vi "Untitled 9 (SubVI).vi"(0 "background \n coincidence counts":dbl, 1 "sigma (mrad) in":dbl, 2 "collimator afstand\n       (mm)":dbl, 3 "alignment correction":dbl, 4 "spleetbreedte\n      (mm)":dbl, 5 "1d - Acar":bool, 6 "all rows":ext[][](array[numeric]), 8 "22Na source radius (mm)":dbl, 9 "stop in":bool, 10 "core width\n   (mrad)":dbl, 11 "stop 4":bool, 12 "fraction core\nannihilations":dbl, 14 "Fermi angle\n   (mrad)":dbl) -> (13 "2d - Acar 4":bool, 15 "2d - Acar 2":bool, 16 "free gas model":cluster{"Y":dbl[], "Y":dbl[]}[](graph), 17 "ZICHT  functie":cluster{"Y":dbl[], "Y":dbl[]}[](graph), 18 "core electrons":cluster{"Y":dbl[], "Y":dbl[]}[](graph), 19 "2d - Acar 3":bool, 20 "output cluster 2":cluster{ext[], ext[]}, 21 "Sum of squared residuals":dbl, 22 "stop 3":bool, 23 "XY Graph 5":cluster{ext[], "Array out":ext[]}[](graph), 24 "XY Graph 4":cluster{ext[], "Array out":ext[]}[](graph), 25 "?":dbl format="%#_3g", 26 "Fermi energy (eV)":dbl format="%#_3g")   [LabVIEW 2013]
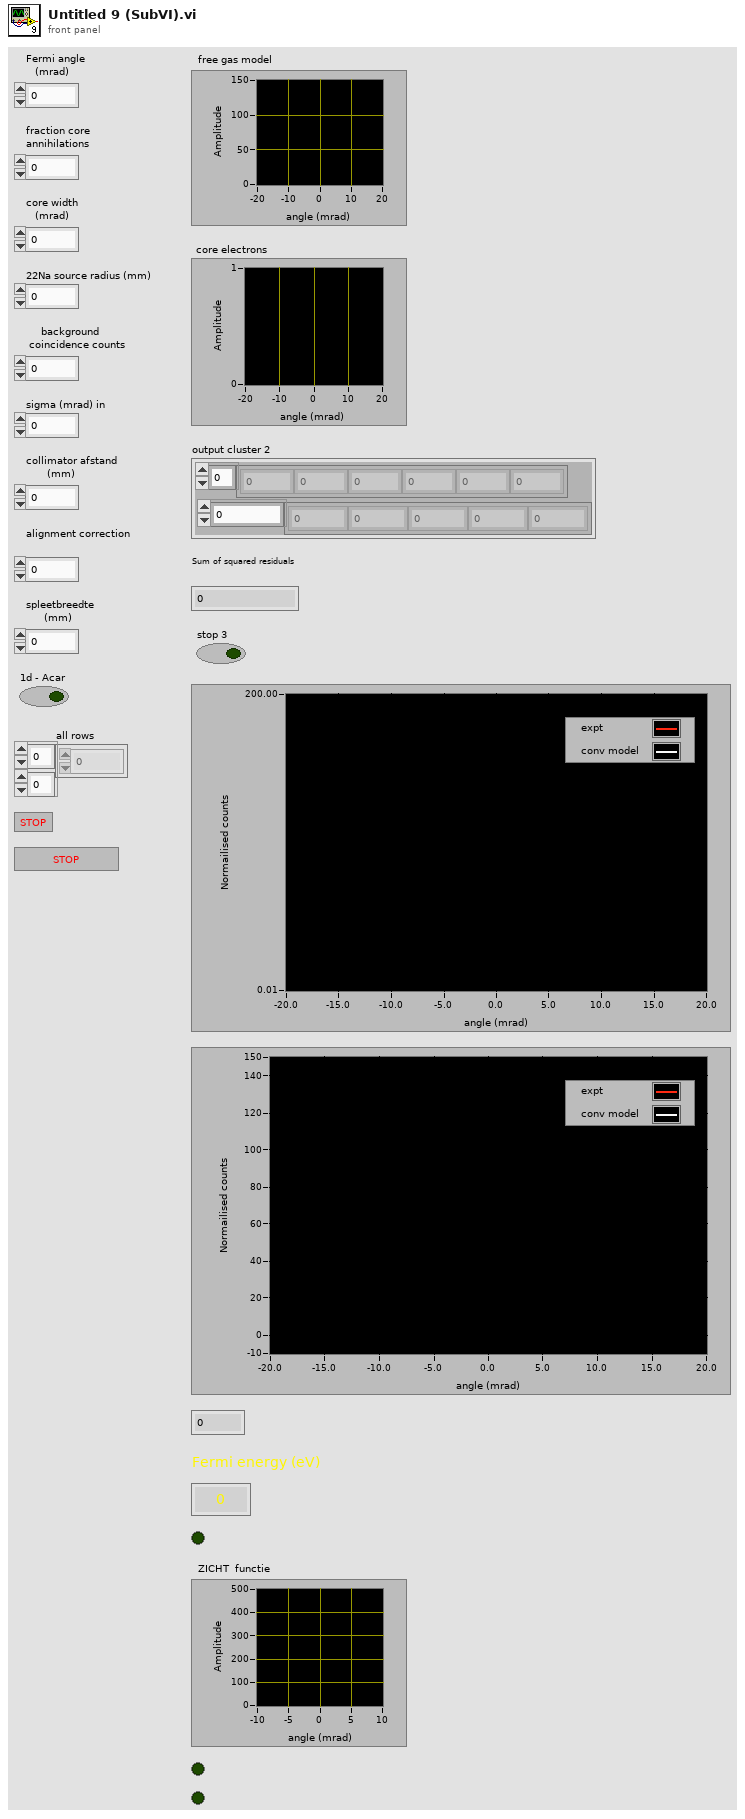
[diagram p1: front panel]
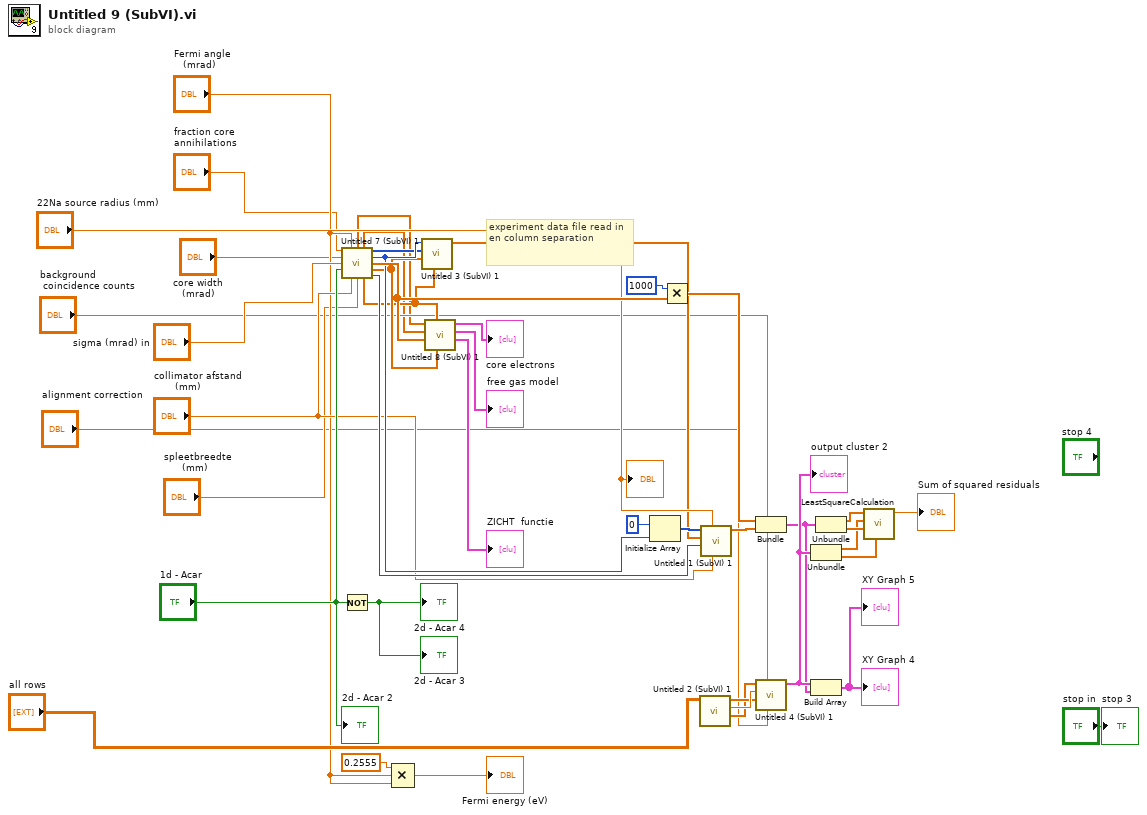
[diagram p0: block diagram]
diagram:
  # "experiment data file read in\nen column separation"
  n1 = call "Untitled 7 (SubVI) 1.vi"("fraction core\nannihilations"="fraction core\nannihilations", "Fermi angle\n   (mrad)"="Fermi angle\n   (mrad)", "core width\n   (mrad)"="core width\n   (mrad)", "sigma (mrad) in"="sigma (mrad) in", "1d - Acar"="1d - Acar", "collimator afstand\n       (mm)"="collimator afstand\n       (mm)", "spleetbreedte\n      (mm)"="spleetbreedte\n      (mm)") -> ("Array 5"=w3:dbl[], "Array 6"=w1:dbl[], "Array 4"=w12:i32[], "Numeric"=w21:i32, "Array"=w31:dbl[], "Array 2"=w14:dbl[], "Array 3"=w13:dbl[], "Numeric 5"=w19:i32)  [unwired: 1 in]
  n2 = Not(x="1d - Acar") -> (.not. x?=→"2d - Acar 3" →"2d - Acar 4":bool)
  n3 = Compound Arithmetic op=MULTIPLY(0.2555, "Fermi angle\n   (mrad)", "Fermi angle\n   (mrad)") -> (→"Fermi energy (eV)":dbl)
  n4 = call "Untitled 3 (SubVI) 1.vi"("Array 3"=w13, "Array in"=w14, "Array 4"=w12, "Numeric"=w21) -> ("Array out"=w22:dbl[])  [unwired: 7 in]
  n5 = call "Untitled 8 (SubVI) 1.vi"("Array 2"=w14, "Array 3"=w13, "Array"=w31, "Array 6"=w1, "Array 5"=w3) -> ("ZICHT  functie"=→"ZICHT  functie":cluster{"Y":dbl[], "Y":dbl[]}[], "free gas model"=→"free gas model":cluster{"Y":dbl[], "Y":dbl[]}[], "core electrons"=→"core electrons":cluster{"Y":dbl[], "Y":dbl[]}[])  [unwired: 4 in]
  n6 = Initialize Array(0, w21) -> (w23:i32[])
  n7 = Multiply(x=1000, y=w31) -> (x*y=w27:dbl[])
  n8 = call "Untitled 2 (SubVI) 1.vi"("all rows"="all rows") -> ("Array 2"=w15:ext[], "Numeric"=w17:ext, "Array"=w16:ext[])  [unwired: 8 in]
  n9 = call "Untitled 1 (SubVI) 1.vi"("collimator afstand\n       (mm)"="collimator afstand\n       (mm)", "22Na source radius (mm)"="22Na source radius (mm)", "Numeric"=w19, "Array 3"=w22, "Array in"=w23) -> ("Array out"=w25:dbl[])  [unwired: 6 in]
  n10 = Bundle(w27, "Array out"=w25) -> (w33:cluster{dbl[], "Array out":dbl[]})  [unwired: 1 in]
  n11 = call "Untitled 4 (SubVI) 1.vi"("alignment correction"="alignment correction", "background \n coincidence counts"="background \n coincidence counts", "Array"=w16, "Numeric"=w17, "Array 2"=w15) -> ("Cluster"=w34:cluster{ext[], ext[]})  [unwired: 6 in]
  "output cluster 2" <- w34
  n12 = Unbundle(w34) -> (w37:ext[], w39:ext[])
  n13 = Build Array(w34, w33) -> (→"XY Graph 4" →"XY Graph 5":cluster{ext[], "Array out":ext[]}[])
  n14 = Unbundle(w33) -> (w36:dbl[], "Array out"=w38:dbl[])
  n15 = call "LeastSquareCalculation.vi"("array 4"=w39, "array 3"=w38, "array 2"=w37, "array"=w36) -> ("Numeric"=→"Sum of squared residuals":dbl)  [unwired: 7 in]
  "?" <- "22Na source radius (mm)"
  "2d - Acar 2" <- "1d - Acar"
  "stop 3" <- "stop in"
